vi "UV_TemplateParam.vi"(7 "R/W (F:read)":bool, 8 "error in":errorcluster, 9 "temp_param":T1(array[cluster]), 10 "Temp_Type":T2 items=["All", "Type 1", "Type 2", "Type 3", "Type 4", "Type 5", "Type 6"], 11 "VISA resource":refnum<visa-resource-name>) -> (0 "error out":errorcluster, 2 "respons":u8[](array[numeric]) format="%.0x", 3 "VISA resource out":refnum<visa-resource-name>, 5 "Err?":bool)   [LabVIEW 8.6]
uses:
  TypeDef/UVLed_func.ctl
  TypeDef/UVLed_TempType.ctl
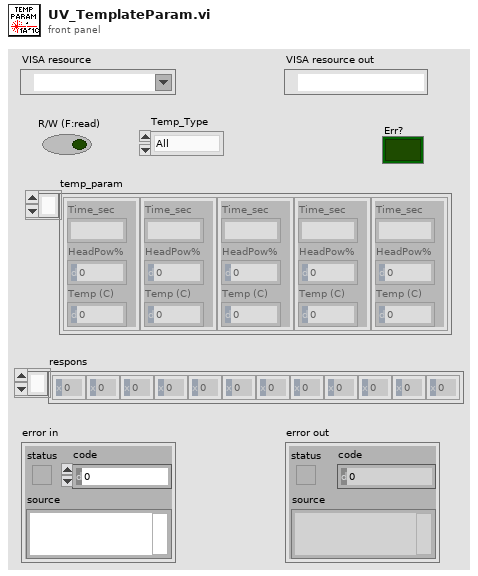
[diagram p1: front panel]
types:
  T1 = cluster{"Time_sec":string, "HeadPow%":i32, "Temp (C)":u8}[]
  T2 = typedef "UVLed_TempType.ctl" = u16
  T3 = typedef "UVLed_func.ctl" = u16
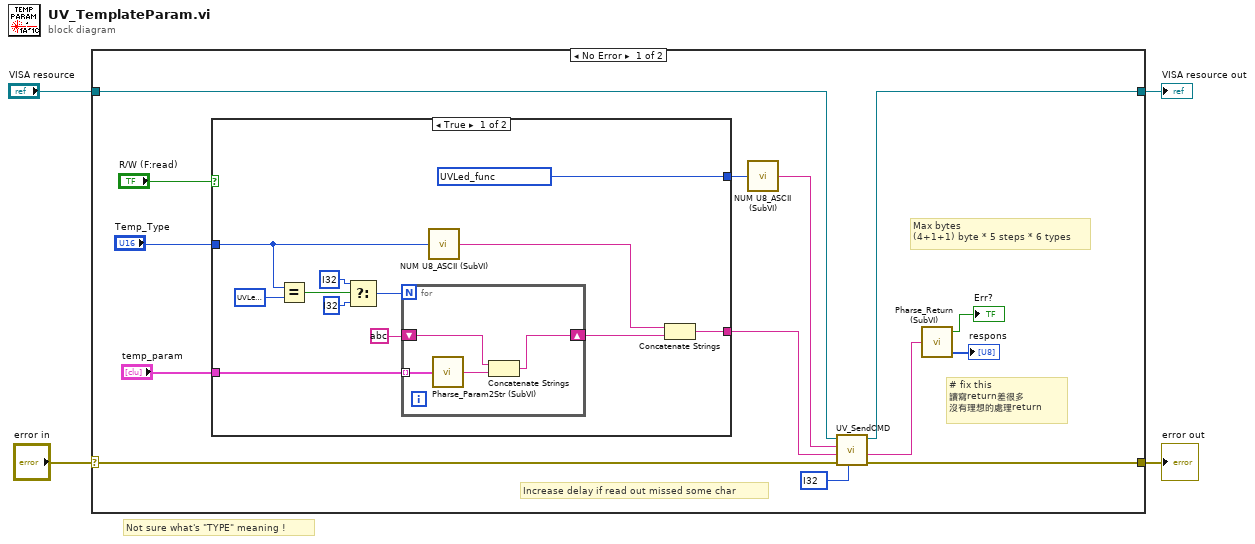
[diagram p0: block diagram]
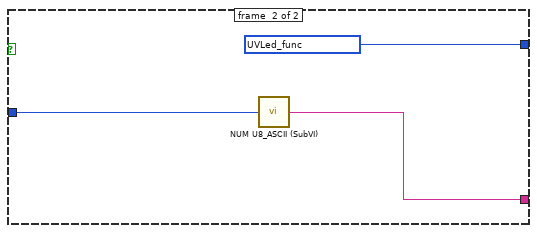
[diagram p2: hidden frame]
diagram:
  # "Not sure what's \"TYPE\" meaning !"
  n1 = case shown="No Error" "error in" {
    selector: "error in" -> [w15 w39]
    tunnel: [w14 w39] -> w3
    tunnel: "VISA resource" -> [w16 w38]
    tunnel: [w12 w38] -> w1
    frame #0 {
      # "Increase delay if read out missed some char"
      # "# fix this\n讀寫return差很多\n沒有理想的處理return"
      # "Max bytes\n(4+1+1) byte * 5 steps * 6 types"
      n2 = case shown="True" "R/W (F:read)" {
        tunnel: [w30 w36] -> w18
        tunnel: [w19 w37] -> w10
        tunnel: "Temp_Type" -> [w22 w35]
        tunnel: "temp_param" -> [w25 _]
        frame #0 {
          w24 = T2 ? items=["All", "Type 1", "Type 2", "Type 3", "Type 4", "Type 5", "Type 6"] ("Temp_Type")
          w30 = T3 ? items=["GetAllStatus", "LightOn", "LightOff", "AllForceOff", "GetMenuChnPara", "SetMenuChnPara", "GetAutoChnPara", "SetAutoChnPara", "GetMenuProTempNo", "SetMenuProTempNo", "GetAutoProTempNo", "SetAutoProTempNo", "GetTemplatePara", "SetTemplatePara", "GetMode", "SetMode"] ("Function")
          n3 = Equal?(x=w22, y=w24) -> (x = y?=w29:bool)
          n4 = Select(t=i32 ?, s=w29, f=i32 ?) -> (s? t:f=w28:i32)
          n5 = for {
            N: w28 -> [_]
            tunnel: w25 -> [w34] mode=indexing
            shift-right: [w31] -> w20
            shift-left: string ? -> [w33]
            n6 = call "Pharse_Param2Str (SubVI).vi"("param"=w34) -> ("param_cmd"=w32:string)
            n7 = Concatenate Strings(w33, w32) -> (w31:string)
          }
          n8 = call "NUM U8_ASCII (SubVI).vi"("Numeric"=w22) -> ("String out"=w21:string)
          n9 = Concatenate Strings(w21, w20) -> (w19:string)
        }
        frame #1 {
          w36 = T3 ? items=["GetAllStatus", "LightOn", "LightOff", "AllForceOff", "GetMenuChnPara", "SetMenuChnPara", "GetAutoChnPara", "SetAutoChnPara", "GetMenuProTempNo", "SetMenuProTempNo", "GetAutoProTempNo", "SetAutoProTempNo", "GetTemplatePara", "SetTemplatePara", "GetMode", "SetMode"] ("Function")
          n10 = call "NUM U8_ASCII (SubVI).vi"("Numeric"=w35) -> ("String out"=w37:string)
        }
      }
      n11 = call "NUM U8_ASCII (SubVI).vi"("Numeric"=w18) -> ("String out"=w17:string)
      n12 = call "UV_SendCMD.vi"("delay(ms)"=i32 ?, "error in"=w15, "value"=w10, "function"=w17, "VISA resource name"=w16) -> ("error out"=w14:errorcluster, "response"=w13:string, "VISA resource name out"=w12:refnum<visa-resource-name>)  [unwired: 4 in]
      n13 = call "Pharse_Return (SubVI).vi"("buffer in"=w13) -> ("byte array"=→"respons":u8[], "Err?"=→"Err?":bool)  [unwired: 2 in, 1 out]
    }
    frame #1 {
    }
  }
  "error out" <- w3
  "VISA resource out" <- w1
